vi "Cache.Create.vi"(8 "error in (no error)":errorcluster, 10 "Transfers":refnum<class "Transfer.lvclass">[](array[class]), 11 "Transfers Groups":refnum<class "Transfer Group.lvclass">[](array[class])) -> (0 "error out":errorcluster, 3 "Cache out":refnum<class "Cache.lvclass">)   [LabVIEW 2017, in "DSF Core.lvlib" / "Cache.lvclass"]
uses:
  Cache.lvclass
  Transfer/Transfer.lvclass
  Transfer/Transfer Group.lvclass
  Cache.lvclass/Cache.ctl
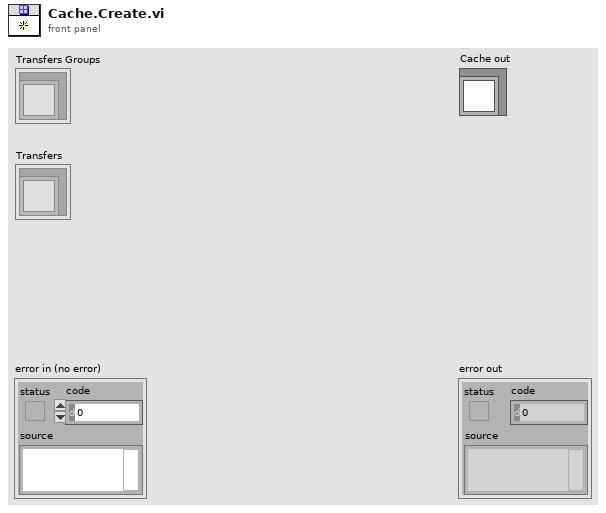
[diagram p1: front panel]
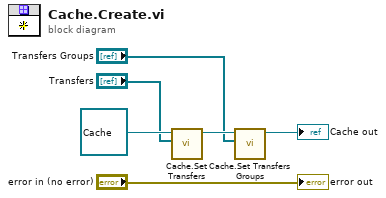
[diagram p0: block diagram]
diagram:
  n1 = call "Cache.Set Transfers.vi"("Transfers"="Transfers", "Cache in"=refnum<class "Cache.lvclass"> refnum) -> ("Cache out"=w4:refnum<class "Cache.lvclass">)  [unwired: 9 in]
  n2 = call "Cache.Set Transfers Groups.vi"("Transfers Groups"="Transfers Groups", "Cache in"=w4) -> ("Cache out"=→"Cache out":refnum<class "Cache.lvclass">)  [unwired: 9 in]
  "error out" <- "error in (no error)"
